vi "test.vi"() -> ()   [LabVIEW 2018]
uses:
  <vilib>/imath/engines/lvmath2/RunTimeEngine/NodeEndStatement/NIMS_NodeEndStatement_Output.vi
  <instcachedir>/0/NIMS_NodeEndStatement_Output_53EC0D466D134D7ABD903AC30B43404B.lvgen/NIMS_NodeEndStatement_Output_53EC0D466D134D7ABD903AC30B43404B_002.vi
  <vilib>/imath/engines/lvmath2/RunTimeEngine/ErrorHandling/NIMS_Finalize Error.vi
panel:
  out "element":dbl[][](array[numeric])
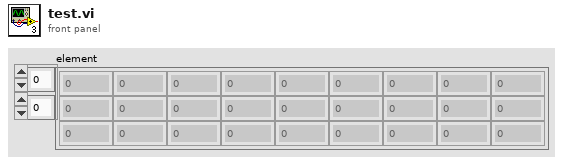
[diagram p1: front panel]
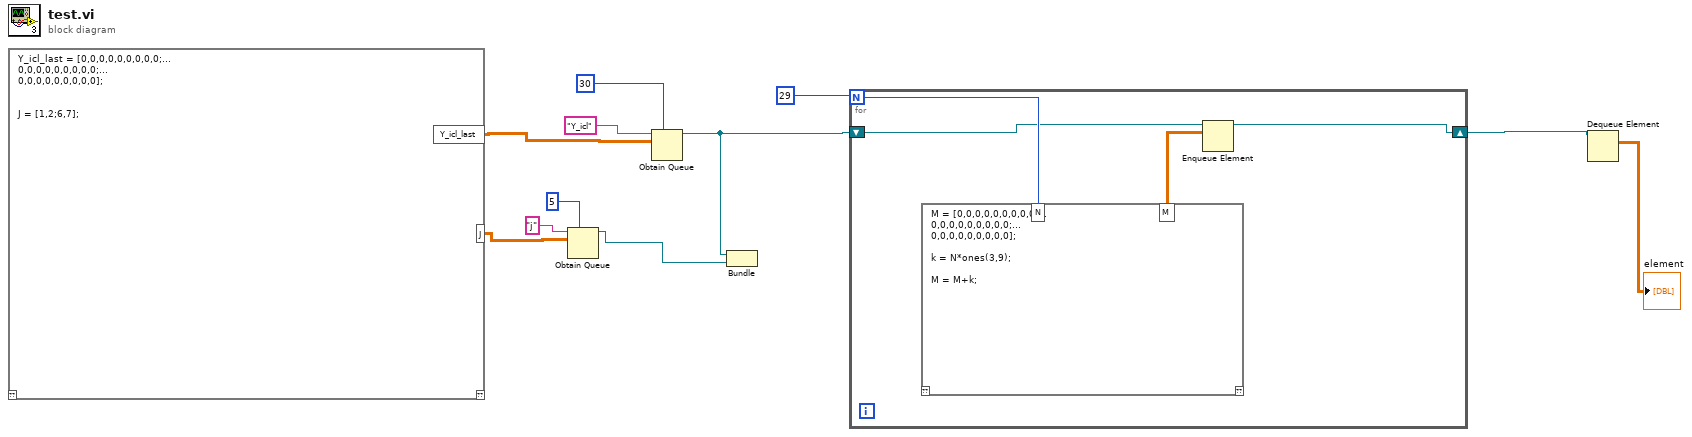
[diagram p0: block diagram]
diagram:
  n1 = mathscript code="Y_icl_last = [0,0,0,0,0,0,0,0,0;...\n0,0,0,0,0,0,0,0,0;...\n0,0,0,0,0,0,0,0,0];\n\n\nJ = [1,2;6,7];"() -> ("Y_icl_last"=w9:dbl[][], "J"=w4:dbl[][])  [unwired: 1 in, 1 out]
  n2 = Obtain Queue(max queue size (-1, unlimited)=5, name (unnamed)="j", element data type=w4) -> (queue out=w2:refnum<queue>)  [unwired: 2 in, 2 out]
  n3 = Obtain Queue(max queue size (-1, unlimited)=30, name (unnamed)="Y_icl", element data type=w9) -> (queue out=w3:refnum<queue>)  [unwired: 2 in, 2 out]
  n4 = Bundle("queue out"=w3, "queue out"=w2) -> ()  [unwired: 1 in, 1 out]
  n5 = for {
    N: 29 -> [w15]
    shift-right: [w12] -> w7
    shift-left: w3 -> [w13]
    n6 = mathscript code="M = [0,0,0,0,0,0,0,0,0;...\n0,0,0,0,0,0,0,0,0;...\n0,0,0,0,0,0,0,0,0];\n\nk = N*ones(3,9);\n\nM = M+k;"("N"=w15) -> ("M"=w14:dbl[][])  [unwired: 1 in, 1 out]
    n7 = Enqueue Element(queue=w13, element=w14) -> (queue out=w12:refnum<queue>)  [unwired: 2 in, 2 out]
  }
  n8 = Dequeue Element(queue=w7) -> (element=→"element":dbl[][])  [unwired: 2 in, 3 out]
